vi "calc zero.vi"(8 "x2":dbl, 9 "t2":dbl, 10 "x1":dbl, 11 "t1":dbl) -> (0 "tcross":dbl)   [LabVIEW 2017]
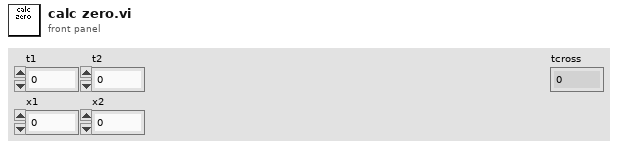
[diagram p1: front panel]
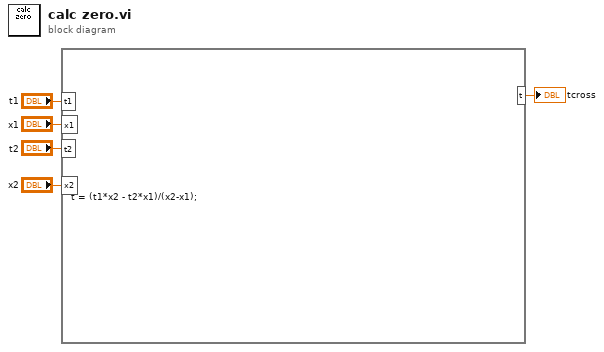
[diagram p0: block diagram]
diagram:
  n1 = formula code="t = (t1*x2 - t2*x1)/(x2-x1);"("t1"="t1", "x1"="x1", "t2"="t2", "x2"="x2") -> ("t"=→"tcross":dbl)
